vi "Build Path.vi"(5 "Subroutine in":refnum<class "Subroutine.lvclass">, 6 "Path Builder":refnum<class "IPath Builder.lvclass">, 7 "Linked List ID":string, 8 "error in (no error)":errorcluster, 11 "Linked List Ref":refnum<data-value>) -> (0 "error out":errorcluster, 2 "Path":path, 3 "Linked List Ref out":refnum<data-value>)   [LabVIEW 2019, in "Test Executive.lvlib" / "Subroutine.lvclass"]
uses:
  <vilib>/gpm_packages/@cs/test-executive/Source/Test Executive/Subroutine/Subroutine.lvclass
  <vilib>/gpm_packages/@cs/linked-list/Source/Linked List/ILinkedList/ILinked List.lvclass
  <vilib>/gpm_packages/@cs/test-executive/Source/Path Builder/IPath Builder/IPath Builder.lvclass
  5b1a0bb9-5619-47ef-ba3e-574aeff7f1ec.vi
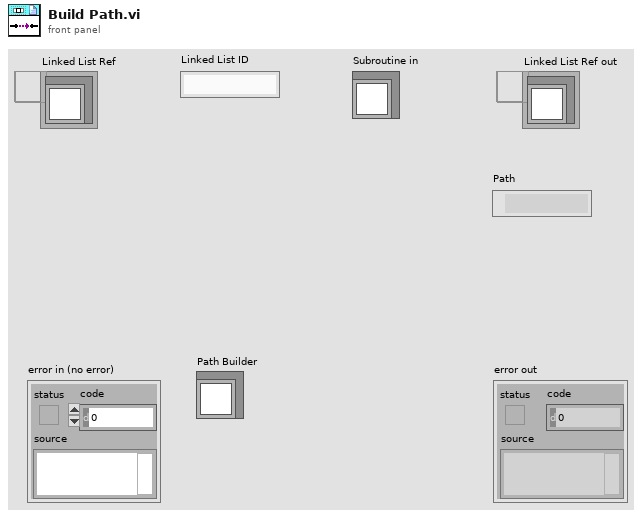
[diagram p1: front panel]
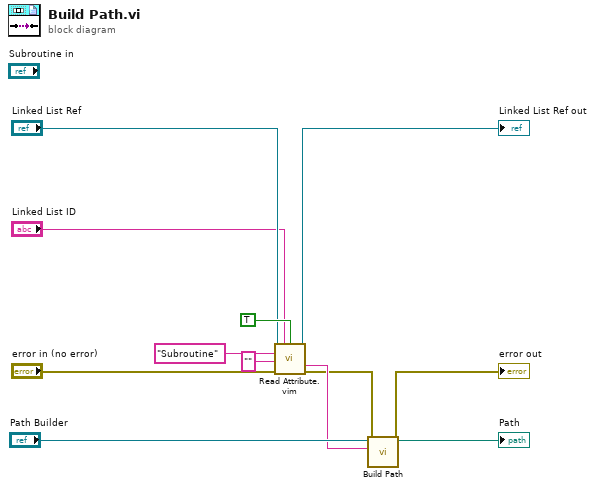
[diagram p0: block diagram]
diagram:
  n1 = call "Read Attribute.vim"("Linked List Ref"="Linked List Ref", "Linked List ID"="Linked List ID", "Include Private?"=TRUE, "Attribute Name"="Subroutine", "Type"="", "error in (no error)"="error in (no error)") -> ("Linked List Ref out"=→"Linked List Ref out":refnum<data-value>, "Attribute"=w4:string, "error out"=w3:errorcluster)  [unwired: 4 in, 3 out]
  n2 = call-dynamic "Build Path.vi"("error in (no error)"=w3, "Path"=w4, "IPath Builder in"="Path Builder") -> ("error out"=→"error out":errorcluster, "Path"=→"Path":path)  [unwired: 7 in]
